vi "Untitled 3.vi"() -> ()   [LabVIEW 2011]
uses:
  <vilib>/Instr/_visa.llb/VISA Set IO Buffer Mask.ctl
  <vilib>/Instr/_visa.llb/VISA Flush IO Buffer Mask.ctl
  <vilib>/Instr/_visa.llb/VISA Configure Serial Port (Instr).vi
panel:
  out "Serial Settings:Number of Bytes at Serial Port":u32
  out "x+y":u32
  out "Numeric 2":i32
  out "Numeric":i32
  out "return count 2":u32
  in  "stop":bool
  out "Position":dbl[](array[numeric]) format="%#_6f"
  out "return count":u32
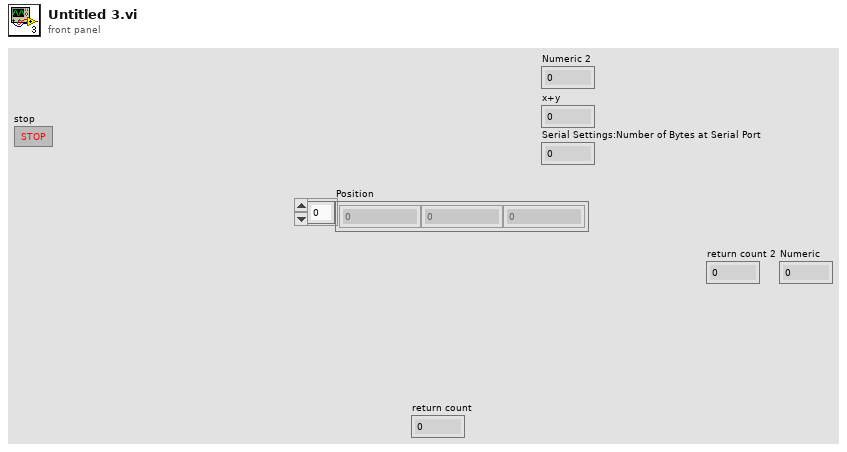
[diagram p1: front panel]
types:
  T1 = typedef "VISA Set IO Buffer Mask.ctl" = u16
  T2 = typedef "VISA Flush IO Buffer Mask.ctl" = u16
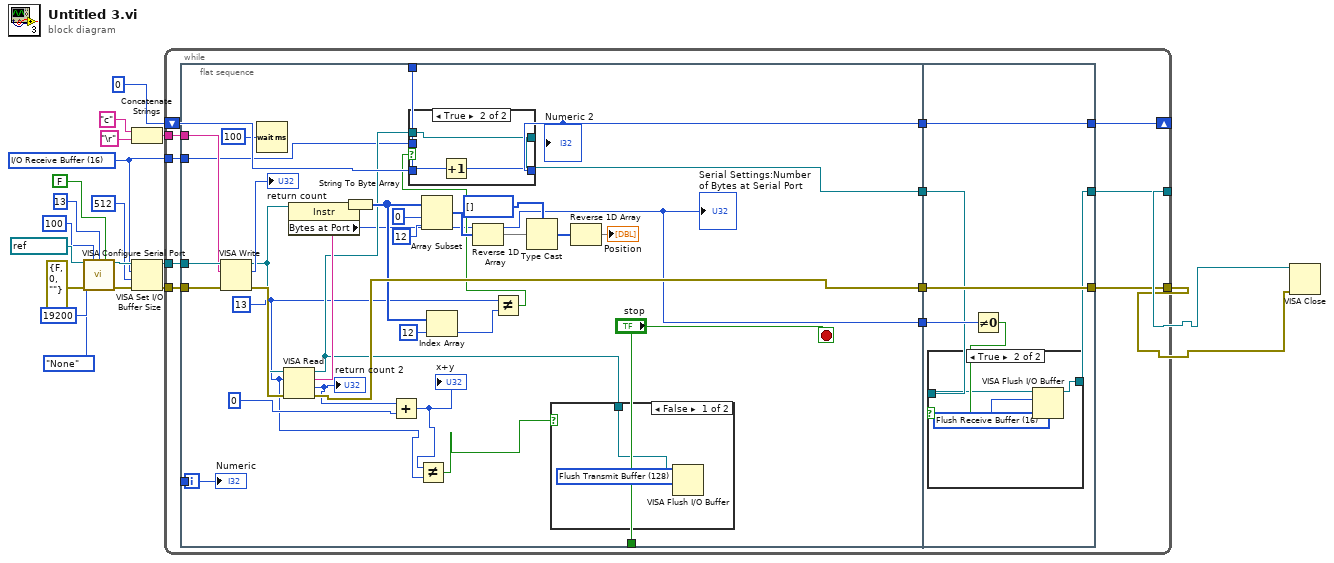
[diagram p0: block diagram]
diagram:
  w5 = T1 16 items=["I/O Receive Buffer"=16, "I/O Transmit Buffer"=32, "I/O Receive and Transmit Buffer"=48] ("Control")
  n1 = call-poly "VISA Configure Serial Port"("VISA resource name"=refnum<visa-resource-name> "COM6", "timeout (10sec)"=u32 100, "termination char\n(0xA = '\\n' = LF)"=u8 13 ("termination char\n(0xA = '\\n' = LF)"), "Enable Termination\nChar (T)"=FALSE ("Enable Termination\nChar (T)"), "baud rate (9600)"=u32 19200, "parity (0:none)"=enum16{"None", "Odd", "Even", "Mark", "Space"}."None", "error in (no error)"=errorcluster {"status"=FALSE, "code"=0, "source"=""}) -> ("VISA resource name out"=w13:refnum<visa-resource-name>, "error out"=w12:errorcluster)  [unwired: 7 in]
  n2 = Concatenate Strings("c" ("string"), "\r" ("write buffer")) -> (w10:string)
  n3 = VISA Set I/O Buffer Size(VISA resource name=w13, mask (16)=w5, size (4096)=u32 512, error in (no error)=w12) -> (VISA resource name out=w11:refnum<visa-resource-name>, error out=w9:errorcluster)
  n4 = while {
    tunnel: [w24] -> w2
    tunnel: [w28] -> w1
    tunnel: w11 -> [w31]
    tunnel: w10 -> [w30]
    tunnel: w9 -> [w29]
    shift-right: [w26] -> _
    shift-left: 0 -> [w27]
    tunnel: w5 -> [w25]
    i -> [w32]
    stop <- w33 stop-if-true
    n5 = flat-sequence {
      tunnel: ["stop"] -> w33
      tunnel: w32 -> [w54]
      tunnel: w31 -> [w53]
      tunnel: w30 -> [w52]
      tunnel: w29 -> [w51]
      tunnel: w27 -> [w45]
      tunnel: w25 -> [w42]
      tunnel: [w50] -> w23
      tunnel: [w44] -> w22
      tunnel: [w41] -> w21
      tunnel: [w38] -> w20
      tunnel: [w74] -> w24
      tunnel: [w78] -> w26
      tunnel: [w79] -> w28
      tunnel: w23 -> [w79]
      tunnel: w22 -> [w78]
      tunnel: w21 -> [w75]
      tunnel: w20 -> [w77]
      frame #0 {
        w35 = 13
        n6 = VISA Write(VISA resource name=w53, write buffer=w52, error in (no error)=w51) -> (VISA resource name out=w39:refnum<visa-resource-name>, return count=→"return count":u32, error out=w65:errorcluster)
        n7 = Wait (ms)(milliseconds to wait=u32 100) -> ()  [unwired: 1 out]
        n8 = VISA Read(VISA resource name=w39, byte count=w35, error in (no error)=w65) -> (VISA resource name out=w43:refnum<visa-resource-name>, read buffer=w59:string, return count=w37:u32, error out=w50:errorcluster)
        "return count 2" <- w37
        n9 = property class="Instr"(reference=w39) -> ("Bytes at Port"=w38:u32)  [unwired: 1 in, 2 out]
        "Serial Settings:Number of Bytes at Serial Port" <- w38
        n10 = String To Byte Array(string=w59) -> (unsigned byte array=w49:u8[])
        n11 = Add(x=w37, y=0) -> (x+y=w36:u32)
        "x+y" <- w36
        n12 = Not Equal?(x=w36, y=w35) -> (x != y?=w34:bool)
        n13 = Array Subset(array=w49, index=0, length=12) -> (w62:u8[])
        n14 = Index Array(array=w49, index=12) -> (element=w47:u8)
        n15 = Reverse 1D Array(array=w62) -> (reversed array=w63:u8[])
        n16 = Not Equal?(x=w35, y=w47) -> (x != y?=w46:bool)
        n17 = case shown="True" w46 {
          tunnel: w45 -> [w70 w73]
          tunnel: [w70 w72] -> w44
          tunnel: w43 -> [w69 w71]
          tunnel: w42 -> [_ _]
          tunnel: [w69 w71] -> w41
          frame False {
          }
          frame True {
            n18 = Increment(x=w73) -> (x+1=w72:i32)
          }
        }
        "Numeric 2" <- w44
        n19 = Type Cast(type=i32[] [], x=w63) -> (*(type *) &x=w64:i32[])
        n20 = case shown="False" w34 {
          tunnel: w43 -> [w68 _]
          frame False {
            w67 = T2 128 items=["Flush Receive Buffer"=16, "Write Transmit Buffer to Device"=32, "Flush Receive Buffer (No I/O)"=64, "Flush Transmit Buffer"=128] ("Mask")
            n21 = VISA Flush I/O Buffer(VISA resource name=w68, mask (16)=w67) -> ()  [unwired: 1 in, 2 out]
          }
          frame True {
          }
        }
        n22 = Reverse 1D Array(array=w64) -> (reversed array=→"Position":i32[])
        "Numeric" <- w54
      }
      frame #1 {
        n23 = Not Equal To 0?(x=w77) -> (x != 0?=w76:bool)
        n24 = case shown="True" w76 {
          tunnel: w75 -> [w80 w83]
          tunnel: [w80 w82] -> w74
          frame False {
          }
          frame True {
            w81 = T2 16 items=["Flush Receive Buffer"=16, "Write Transmit Buffer to Device"=32, "Flush Receive Buffer (No I/O)"=64, "Flush Transmit Buffer"=128] ("Mask")
            n25 = VISA Flush I/O Buffer(VISA resource name=w83, mask (16)=w81) -> (VISA resource name out=w82:refnum<visa-resource-name>)  [unwired: 1 in, 1 out]
          }
        }
      }
    }
  }
  n26 = VISA Close(VISA resource name=w2, error in (no error)=w1) -> ()  [unwired: 1 out]
